vi "Lab 1 (Thermometer).vi"() -> ()   [LabVIEW 2020]
panel:
  out "Warning":bool
  out "Mode":string
  in  "Switch":bool
  out "Temprature":dbl
  in  "Real World Thermometer C":dbl(slide) scale=0.0..100.0
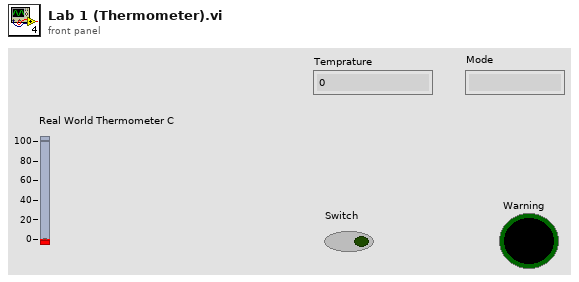
[diagram p1: front panel]
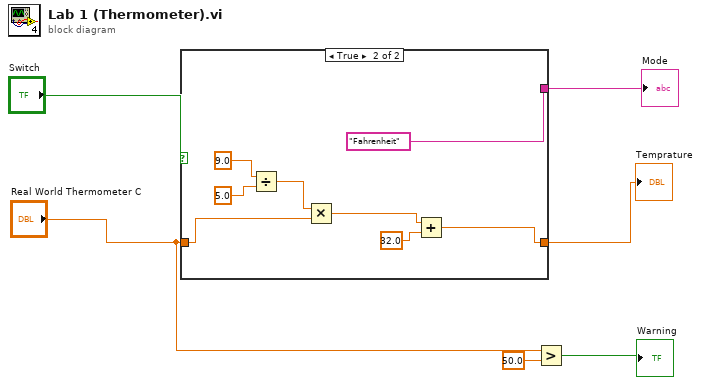
[diagram p0: block diagram]
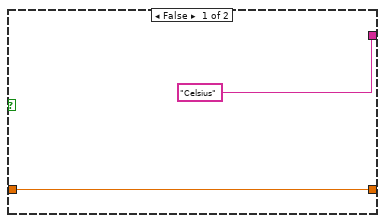
[diagram p2: hidden frame]
diagram:
  n1 = case shown="True" "Switch" {
    tunnel: ["Celsius" "Fahrenheit"] -> w5
    tunnel: "Real World Thermometer C" -> [w7 w12]
    tunnel: [w7 w9] -> w4
    frame False {
    }
    frame True {
      n2 = Divide(x=9.0, y=5.0) -> (x/y=w13:dbl)
      n3 = Multiply(x=w13, y=w12) -> (x*y=w10:dbl)
      n4 = Add(x=w10, y=32.0) -> (x+y=w9:dbl)
    }
  }
  "Temprature" <- w4
  "Mode" <- w5
  n5 = Greater?(x="Real World Thermometer C", y=50.0) -> (0:→"Warning":bool)
